vi "ALTS-2015 Check forTest Result same as Previous Test.vi"(8 "error in":errorcluster, 10 "Current Test Result":string[][](array[string]), 11 "Station Enum":T1) -> (0 "error out":errorcluster, 1 "Test Result":string[][](array[string]), 2 "Result Status":string, 3 "Same as Previous Test Result?":bool)   [LabVIEW 2013]
doc: "Copyright © 2005, Soliton Technologies.\nAll rights reserved."
uses:
  Controls/ALTS-2015 Station Cluster.ctl
  Controls/ALTS-2015 Read Write Cluster Last Saved Results Data cluster.ctl
panel:
  in  "Station Enum":T1
  # "Dont delete this Control. Its Property Nodes are used"
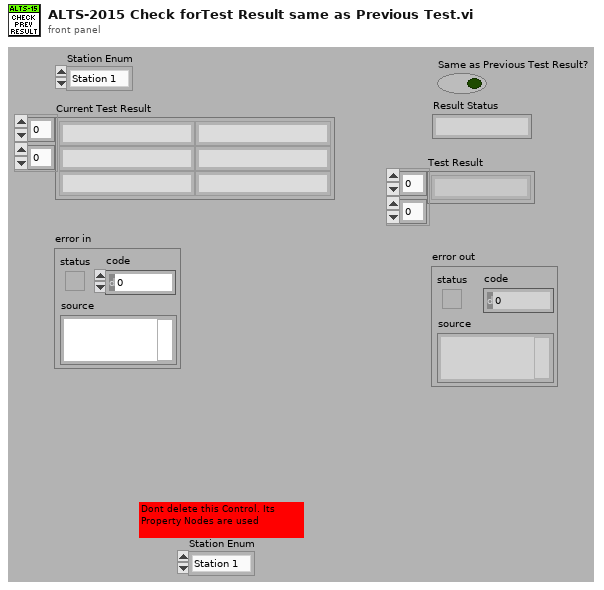
[diagram p1: front panel]
types:
  T1 = typedef "ALTS-2015 Station Cluster.ctl" = enum16{"Station 1", "Station 2", "Station 3", "Station 4"}
  T2 = typedef "ALTS-2015 Read Write Cluster Last Saved Results Data cluster.ctl" = cluster{"Array":string[][][]}
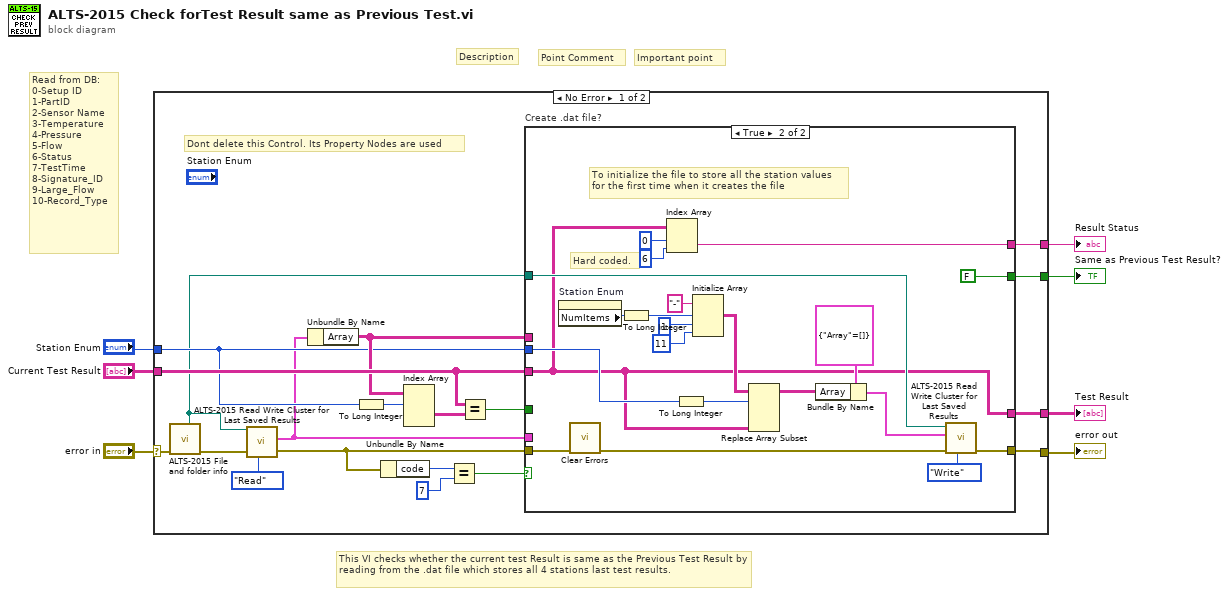
[diagram p0: block diagram]
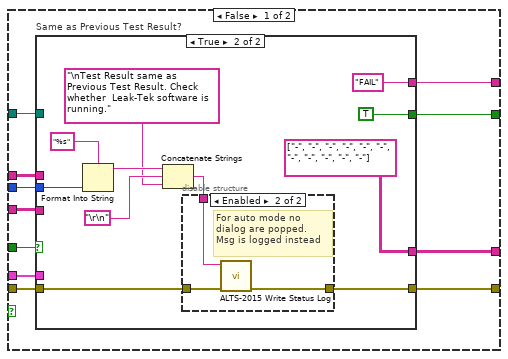
[diagram p2: hidden frame]
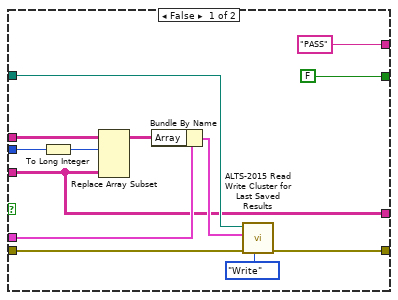
[diagram p3: hidden frame]
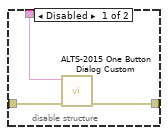
[diagram p4: hidden frame]
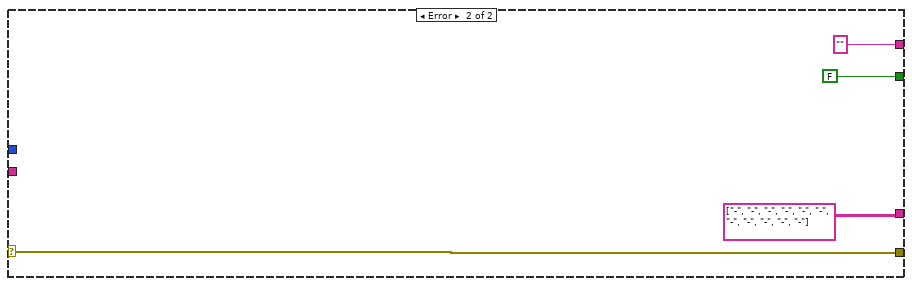
[diagram p5: hidden frame]
diagram:
  # "Read from DB:\n0-Setup ID\n1-PartID\n2-Sensor Name\n3-Temperature\n4-Pressure\n5-Flow\n6-Status\n7-TestTime\n8-Signature_ID\n9-Large_Flow\n10-Record_Type"
  # "This VI checks whether the current test Result is same as the Previous Test Result by reading from the .dat file which stores all 4 stations last test results."
  # "Point Comment"
  # "Important point"
  # "Description"
  n1 = case shown="No Error" "error in" {
    selector: "error in" -> [w20 w92]
    tunnel: [w21 w92] -> w6
    tunnel: "Station Enum" -> [w22 _]
    tunnel: "Current Test Result" -> [w24 _]
    tunnel: [w17 FALSE ("Same as Previous Test Result?")] -> w3
    tunnel: [w16 ""] -> w2
    tunnel: [w15 string[][] [["-", "-", "-", "-", "-", "-", "-", "-", "-", "-", "-"]] ("Current Test Result")] -> w1
    frame No Error {
      # "Dont delete this Control. Its Property Nodes are used"
      n2 = call "ALTS-2015 File and folder info.vi"("error in (no error)"=w20) -> ("error out"=w19:errorcluster, "ALTS Last Test Results File"=w8:path)  [unwired: 2 in, 7 out]
      n3 = call "ALTS-2015 Read Write Cluster for Last Saved Results.vi"("Option"=enum16{"Read", "Write"}."Read", "error in (no error)"=w19, "File path"=w8) -> ("error out"=w14:errorcluster, "Cluster Out"=w18:T2)  [unwired: 6 in, 1 out]
      n4 = Unbundle By Name(w18) -> ("Array"=w23:string[][][])
      n5 = To Long Integer(number=w22) -> (32bit integer=w9:i32)
      n6 = Unbundle By Name(w14) -> ("code"=w13:i32)
      n7 = Index Array(array=w23, index (dim 0)=w9) -> (element=w25:string[][])  [unwired: 2 in]
      n8 = Equal?(x=w13, y=7) -> (x = y?=w11:bool)
      n9 = Equal?(x=w24, y=w25) -> (x = y?=w10:bool)
      n10 = case "Create .dat file?" shown="True" w11 {
        tunnel: w10 -> [w37 _]
        tunnel: w24 -> [w36 w70]
        tunnel: w23 -> [w35 _]
        tunnel: w22 -> [w34 w72]
        tunnel: w14 -> [w33 w74]
        tunnel: [w32 w80] -> w21
        tunnel: w8 -> [w31 w75]
        tunnel: w18 -> [w30 _]
        tunnel: [w29 FALSE ("Same as Previous Test Result?")] -> w17
        tunnel: [w28 w76] -> w16
        tunnel: [w27 w70] -> w15
        frame False {
          n11 = case "Same as Previous Test Result?" shown="True" w37 {
            tunnel: w36 -> [w41 _]
            tunnel: w35 -> [w49 _]
            tunnel: w34 -> [w48 w56]
            tunnel: w30 -> [w47 _]
            tunnel: w33 -> [w40 w61]
            tunnel: [w39 w60] -> w32
            tunnel: w31 -> [w45 _]
            tunnel: [FALSE ("Same as Previous Test Result?") TRUE ("Same as Previous Test Result?")] -> w29
            tunnel: ["PASS" "FAIL"] -> w28
            tunnel: [w41 string[][] [["-", "-", "-", "-", "-", "-", "-", "-", "-", "-", "-"]] ("Current Test Result")] -> w27
            frame False {
              n12 = To Long Integer(number=w48) -> (32bit integer=w38:i32)
              n13 = Replace Array Subset(array=w49, new element=w41, index (dim 0)=w38) -> (w46:string[][][])  [unwired: 2 in]
              n14 = Bundle By Name(cluster=w47, "Array"=w46) -> (w44:T2)
              n15 = call "ALTS-2015 Read Write Cluster for Last Saved Results.vi"("Option"=enum16{"Read", "Write"}."Write", "error in (no error)"=w40, "Cluster In"=w44, "File path"=w45) -> ("error out"=w39:errorcluster)  [unwired: 5 in, 2 out]
            }
            frame True {
              n16 = Format Into String(format string="%s", w56) -> (resulting string=w54:string)  [unwired: 2 in, 1 out]
              n17 = Concatenate Strings(w54, "\r\n", "\nTest Result same as Previous Test Result. Check whether  Leak-Tek software is running." ("message")) -> (w51:string)
              n18 = disable-structure shown="Enabled" {
                disable-tunnel: w61 -> [w64 w67]
                disable-tunnel: [w63 w66] -> w60
                disable-tunnel: w51 -> [w62 w65]
                frame Disabled {
                  n19 = call "ALTS-2015 One Button Dialog Custom.vi"("Error in"=w64, "Message in"=w62) -> ("Error out"=w63:errorcluster)  [unwired: 8 in, 1 out]
                }
                frame Enabled {
                  # "For auto mode no\ndialog are popped.\nMsg is logged instead"
                  n20 = call "ALTS-2015 Write Status Log.vi"("error in (no error)"=w67, "Status Input"=w65) -> ("error out"=w66:errorcluster)  [unwired: 9 in]
                }
              }
            }
          }
        }
        frame True {
          # "Hard coded."
          # "To initialize the file to store all the station values \nfor the first time when it creates the file"
          n21 = property on="Station Enum" class="Enum (strict)"() -> ("NumItems"=w85:u32)  [unwired: 2 in, 2 out]
          n22 = call <vilib>:"Clear Errors.vi"("error in (no error)"=w74) -> ("error out"=w73:errorcluster)  [unwired: 6 in]
          n23 = To Long Integer(number=w85) -> (32bit integer=w84:i32)
          n24 = Index Array(array=w70, index (row)=0, index (col)=6 ("disabled index (col)")) -> (element=w76:string)
          n25 = To Long Integer(number=w72) -> (32bit integer=w68:i32)
          n26 = Initialize Array("-" ("Test Result"), w84, 1 ("dimension size"), 11 ("dimension size")) -> (w71:string[][][])
          n27 = Replace Array Subset(array=w71, new element=w70, index (dim 0)=w68) -> (w69:string[][][])  [unwired: 2 in]
          n28 = Bundle By Name(cluster=T2 {"Array"=[]} ("Cluster In"), "Array"=w69) -> (w87:T2)
          n29 = call "ALTS-2015 Read Write Cluster for Last Saved Results.vi"("Option"=enum16{"Read", "Write"}."Write", "error in (no error)"=w73, "Cluster In"=w87, "File path"=w75) -> ("error out"=w80:errorcluster)  [unwired: 5 in, 2 out]
        }
      }
    }
    frame Error {
    }
  }
  "error out" <- w6
  "Same as Previous Test Result?" <- w3
  "Result Status" <- w2
  "Test Result" <- w1
